vi "GetPumpHandle.vi"(0 "object in":refnum<class "CetoniPump.lvclass">, 5 "error in (no error)":errorcluster) -> (14 "object out":refnum<class "CetoniPump.lvclass">, 15 "Pump handle":i64, 19 "error out":errorcluster)   [LabVIEW 2024, in "CetoniPump.lvclass"]
uses:
  CetoniPump.lvclass
  CetoniPump.lvclass/CetoniPump.ctl
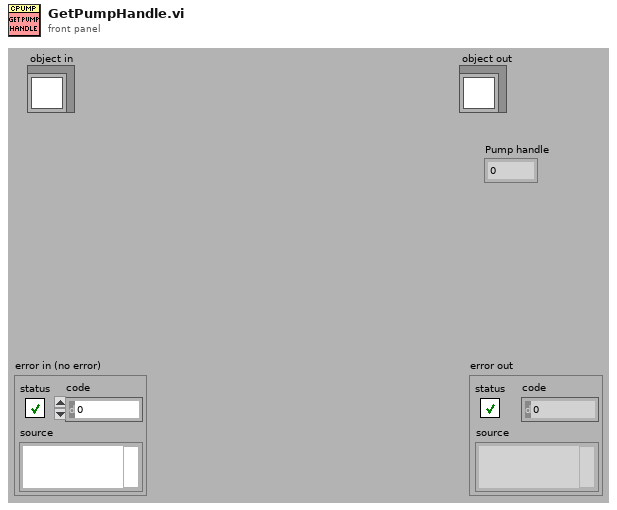
[diagram p1: front panel]
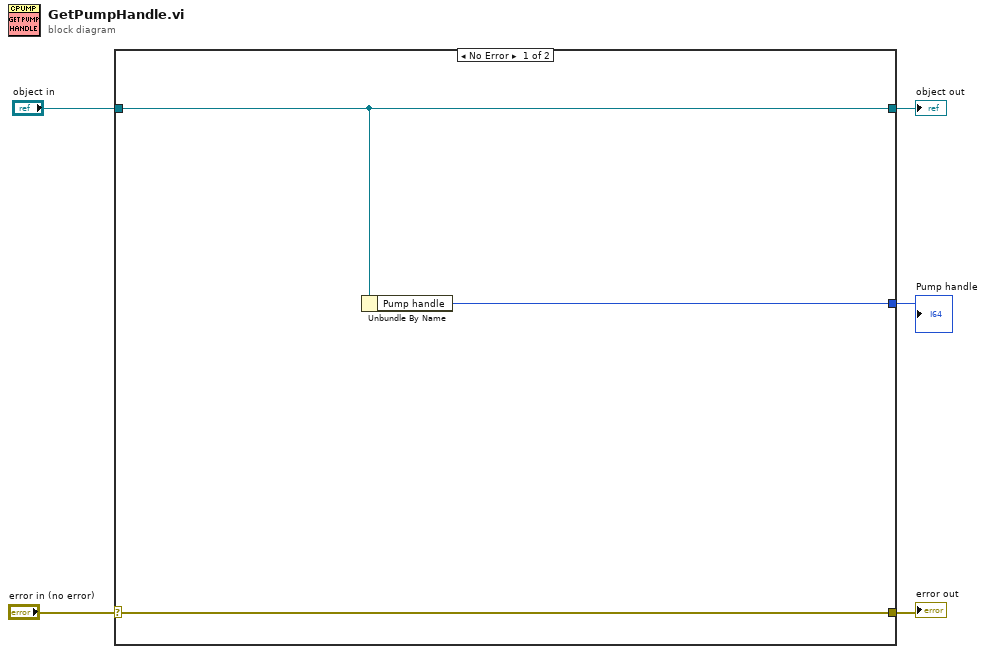
[diagram p0: block diagram]
diagram:
  n1 = case shown="No Error" "error in (no error)" {
    selector: "error in (no error)" -> [w7 w10]
    tunnel: [w7 w10] -> w4
    tunnel: [w6 w9] -> w2
    tunnel: "object in" -> [w6 w9]
    tunnel: [w8 _] -> w1
    frame No Error {
      n2 = Unbundle By Name(w6) -> ("Pump handle"=w8:i64)
    }
    frame Error {
    }
  }
  "error out" <- w4
  "object out" <- w2
  "Pump handle" <- w1
